vi "Indexer PID.vi"() -> ()   [LabVIEW 2011]
uses:
  PID Set Points.vi
  <vilib>/addons/control/pid/pid.llb/PID (DBL).vi
  <vilib>/addons/control/pid/NI_PID_pid.lvlib
panel:
  out "Shootoer RPM":cluster{dbl, dbl, dbl[]}(graph)
  out "Encoder Speed":dbl
  in  "D":dbl
  in  "I":dbl
  out "RPM Error":dbl
  out "Encoder Set Speed":dbl
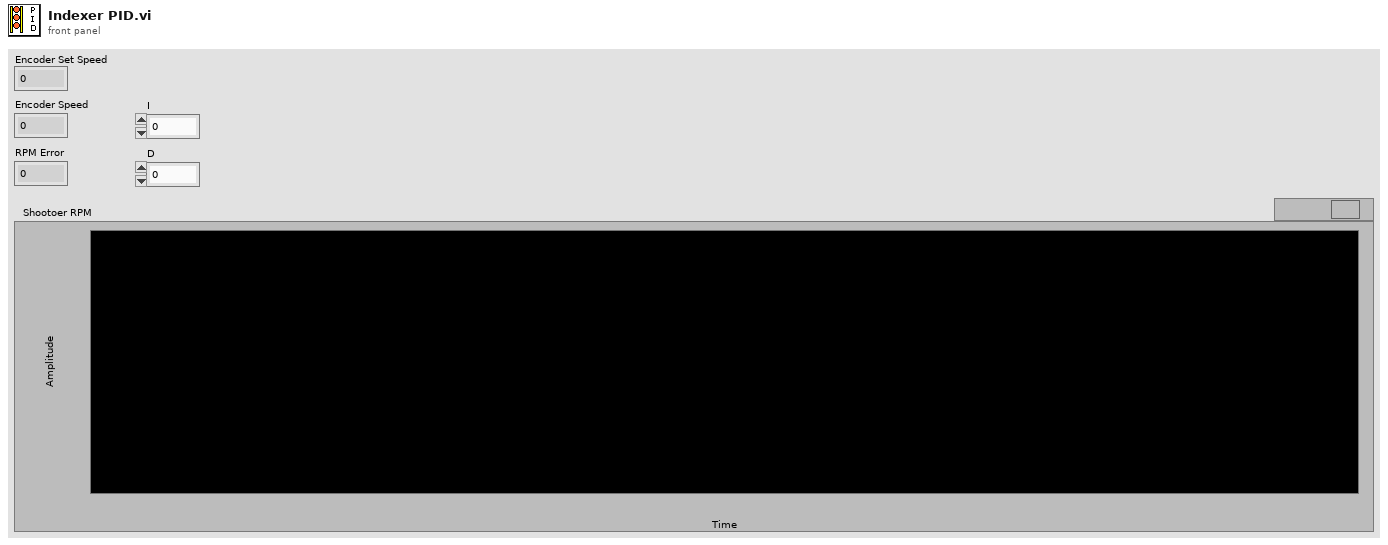
[diagram p1: front panel]
types:
  T1 = typedef "WPI_EncoderDevRef.ctl" = cluster{"DevStatus":errorcluster, "EncoderIndex":T2, "CounterIndex":T3, "DistancePerCount":dbl, "Decoding Type":T4}
  T2 = typedef "FPGA_EncoderIdx.ctl" = enum8{"Enc 0", "Enc 1", "Enc 2", "Enc 3", "Invalid"}
  T3 = typedef "FPGA_CounterCtrSystemIndex.ctl" = enum8{"Ctr 0", "Ctr 1", "Ctr 2", "Ctr 3", "Ctr 4", "Ctr 5", "Ctr 6", "Ctr 7", "Invalid"}
  T4 = typedef "WPI_EncoderType.ctl" = enum16{"1x", "2x", "4x"}
  T5 = typedef "WPI_MotorControlDeviceRef.ctl" = cluster{"DeviceStatus":errorcluster, "Type":enum16{"PWM", "CAN"}, "PWM":cluster{"Digital Module":T6, "PWM Channel":T7, "DeadBand":T8}, "CAN":cluster{"Device Number":u8, "Control Mode":T9, "Semaphore":T10, "Max Vout":dbl}, "Invert":bool, "TransformRef":T11, "InvTransformRef":T11}
  T6 = typedef "FPGA_TypedefDigitalModule.ctl" = enum16{"Digital Module 1", "Digital Module 2"}
  T7 = typedef "FPGA_DIOPWMChannel.ctl" = enum8{"PWM 1", "PWM 2", "PWM 3", "PWM 4", "PWM 5", "PWM 6", "PWM 7", "PWM 8", "PWM 9", "PWM 10", "Invalid"}
  T8 = typedef "WPI_PWMDeadband.ctl" = cluster{"Name":string, "maxPositivePwm":i32, "minPositivePwm":i32, "centerPwm":i32, "maxNegativePwm":i32, "minNegativePwm":i32, "angularRange":u16}
  T9 = typedef "WPI_CANJaguar_ControlMode.ctl" = enum8{"Percent VBus", "Current", "Speed", "Position", "Voltage"}
  T10 = typedef "Semaphore RefNum" = refnum<k1>
  T11 = typedef "WPI_PWMTransform_ConPane.ctl" = refnum<vi>
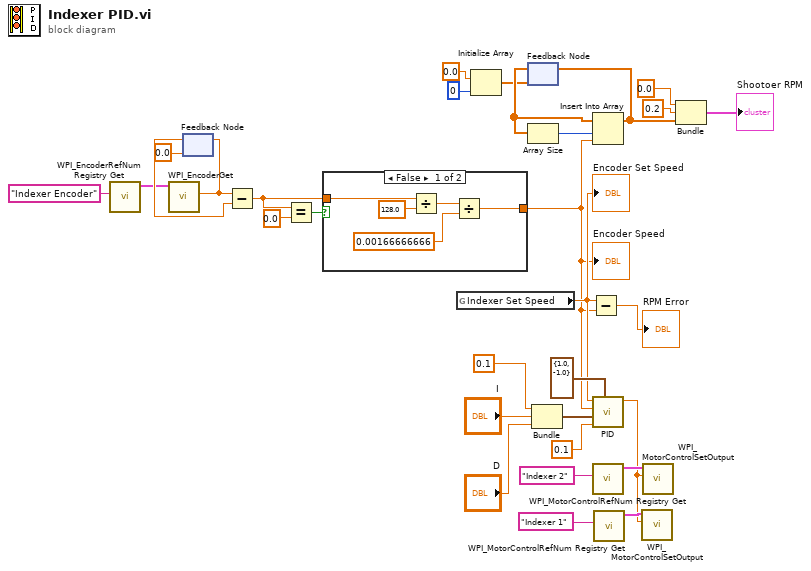
[diagram p0: block diagram]
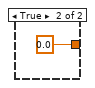
[diagram p2: hidden frame]
diagram:
  n1 = call <vilib>:"WPI_EncoderRefNum Registry Get.vi"("refnum name"="Indexer Encoder") -> ("EncoderDevRef"=w4:T1)  [unwired: 9 in, 1 out]
  n2 = call <vilib>:"WPI_EncoderGet.vi"("EncoderDevRef"=w4) -> ("Distance"=w9:dbl)  [unwired: 5 in, 5 out]
  n3 = feedback #1(0.0) -> (w12:dbl)
  n4 = feedback-in #1(w9) -> ()
  n5 = Subtract(x=w9, y=w12) -> (x-y=w6:dbl)
  n6 = Equal?(x=w6, y=0.0) -> (x = y?=w7:bool)
  n7 = case shown="False" w7 {
    tunnel: [w33 0.0] -> w2
    tunnel: w6 -> [w32 _]
    frame False {
      n8 = Divide(x=w32, y=128.0) -> (x/y=w35:dbl)
      n9 = Divide(x=w35, y=0.00166666666) -> (x/y=w33:dbl)
    }
    frame True {
    }
  }
  "Encoder Speed" <- w2
  n10 = global read "PID Set Points.vi" "Indexer Set Speed"() -> (w3:dbl)
  "Encoder Set Speed" <- w3
  n11 = Initialize Array(0.0 ("element"), 0 ("dimension size")) -> (w15:dbl[])
  n12 = feedback #2(w15) -> (w16:dbl[])
  n13 = Array Size(array=w16) -> (size(s)=w17:i32)
  n14 = Bundle(0.1, "I"="I", "D"="D") -> (w28:cluster{dbl, "I":dbl, "D":dbl})  [unwired: 1 in]
  n15 = Subtract(x=w3, y=w2) -> (x-y=→"RPM Error":dbl)
  n16 = Insert Into Array(array=w16, index=w17, new element=w2) -> (w20:dbl[])
  n17 = feedback-in #2(w20) -> ()
  n18 = call-poly <vilib>:"PID.vi"("output range"=cluster{"output high":dbl, "output low":dbl} {"output high"=1.0, "output low"=-1.0}, "dt (s)"=0.1, "PID gains"=w28, "process variable"=w2, "setpoint"=w3) -> ("output"=w21:dbl)  [unwired: 5 in, 1 out]
  n19 = call <vilib>:"WPI_MotorControlRefNum Registry Get.vi"("refnum name"="Indexer 2") -> ("MotorControlDevRef"=w23:T5)  [unwired: 9 in, 1 out]
  n20 = call <vilib>:"WPI_MotorControlRefNum Registry Get.vi"("refnum name"="Indexer 1") -> ("MotorControlDevRef"=w24:T5)  [unwired: 9 in, 1 out]
  n21 = call <vilib>:"WPI_MotorControlSetOutput.vi"("Output"=w21, "MotorControlDevRef"=w24) -> ()  [unwired: 8 in, 2 out]
  n22 = call <vilib>:"WPI_MotorControlSetOutput.vi"("Output"=w21, "MotorControlDevRef"=w23) -> ()  [unwired: 8 in, 2 out]
  n23 = Bundle(0.0, 0.2, w20) -> (→"Shootoer RPM":cluster{dbl, dbl, dbl[]})  [unwired: 1 in]
